vi "Group 1-Character Tokens.vi"(11 "Array":string[](array[string])) -> (3 "Grouped Tokens":string[](array[string]))   [LabVIEW 2020]
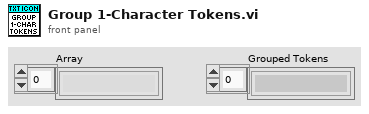
[diagram p1: front panel]
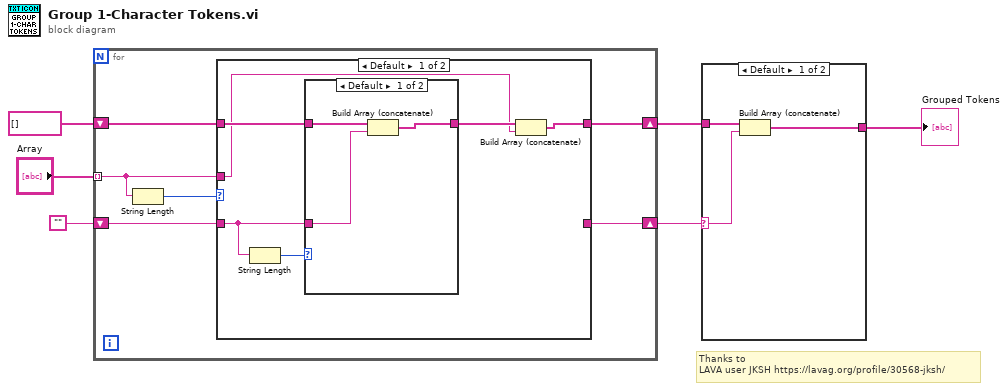
[diagram p0: block diagram]
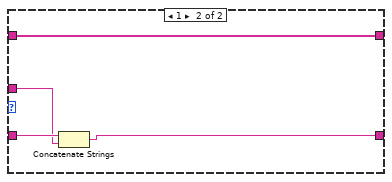
[diagram p4: hidden frame]
diagram:
  # "Thanks to\nLAVA user JKSH https://lavag.org/profile/30568-jksh/"
  n1 = for {
    tunnel: "Array" -> [w10] mode=indexing
    shift-right: [w7] -> w3
    shift-left: "" -> [w11]
    shift-right: [w9] -> w2
    shift-left: string[] [] ("Array") -> [w8]
    n2 = String Length(string=w10) -> (length=w12:i32)
    n3 = case shown="Default" w12 {
      tunnel: w11 -> [w17 w26]
      tunnel: w10 -> [w14 w25]
      tunnel: [w13 w24] -> w9
      tunnel: w8 -> [w16 w24]
      tunnel: [_ w23] -> w7
      frame Default {
        n4 = String Length(string=w17) -> (length=w18:i32)
        n5 = case shown="Default" w18 {
          tunnel: w17 -> [w20 _]
          tunnel: w16 -> [w21 w22]
          tunnel: [w19 w22] -> w15
          frame Default {
            n6 = Build Array (concatenate)(w21, w20) -> (w19:string[])
          }
          frame 0 {
          }
        }
        n7 = Build Array (concatenate)(w15, w14) -> (w13:string[])
      }
      frame 1 {
        n8 = Concatenate Strings(w26, w25) -> (w23:string)
      }
    }
  }
  n9 = case shown="Default" w3 {
    selector: w3 -> [w28 _]
    tunnel: w2 -> [w29 w30]
    tunnel: [w27 w30] -> w1
    frame Default {
      n10 = Build Array (concatenate)(w29, w28) -> (w27:string[])
    }
    frame "" {
    }
  }
  "Grouped Tokens" <- w1
